vi "Set Target.vi"(6 "Axis":T1, 8 "error in (no error)":errorcluster, 9 "Target Rate Limit (T/min)":dbl, 10 "Target Field (T)":dbl[](array[numeric]), 11 "Instrument.VRM in":refnum<class "Instrument.OxfordVRM.lvclass">) -> (0 "error out":errorcluster, 2 "Response":string, 3 "Instrument.VRM out":refnum<class "Instrument.OxfordVRM.lvclass">)   [LabVIEW 2019, in "Instrument.OxfordVRM.lvclass"]
uses:
  Instrument.OxfordVRM.lvclass
  C:/Program Files (x86)/National Instruments/LabVIEW 2019/user.lib/LevyLab/Instrument Framework/SMOs/Instrument/Instrument.lvclass
  Typedefs/VRM Magnet Axis--Enum.ctl
  Typedefs/VRM Targets--Cluster.ctl
  Typedefs/Instrument.VRM.Commands-enum.ctl
  <userlib>/LevyLab/Instrument Framework/SMOs/Instrument/Instrument.lvclass/Instrument.ctl
  7bfbc778-14e2-498e-a779-e48ab3b8e301.vi
  7bfbc778-14e2-498e-a779-e48ab3b8e301.vi/26948dbf-a008-4a5f-8001-90938f97f5fa.vi
  7bfbc778-14e2-498e-a779-e48ab3b8e301.vi/26948dbf-a008-4a5f-8001-90938f97f5fa.vi/85d252fc-3981-4b1f-8816-d182b3c15b0a.vi
  <userlib>/LevyLab/Instrument Framework/SMOs/Instrument/API/Send and Receive.vi
  7bfbc778-14e2-498e-a779-e48ab3b8e301.vi/26948dbf-a008-4a5f-8001-90938f97f5fa.vi/d50f4601-6038-4c2c-b17e-43f1826cda29.vi
  <userlib>/LevyLab/Instrument Framework/SMOs/Instrument/Private/Get Client Type.vi
  7bfbc778-14e2-498e-a779-e48ab3b8e301.vi/26948dbf-a008-4a5f-8001-90938f97f5fa.vi/85d252fc-3981-4b1f-8816-d182b3c15b0a.vi/89440307-fee3-4c08-8f1d-a2867f85d077.vi
  7bfbc778-14e2-498e-a779-e48ab3b8e301.vi/26948dbf-a008-4a5f-8001-90938f97f5fa.vi/85d252fc-3981-4b1f-8816-d182b3c15b0a.vi/71707775-4b93-4dc6-a632-e85984a01861.vi
  7bfbc778-14e2-498e-a779-e48ab3b8e301.vi/26948dbf-a008-4a5f-8001-90938f97f5fa.vi/d50f4601-6038-4c2c-b17e-43f1826cda29.vi/ef93c44c-7e4a-41bd-a109-24ce89437007.vi
  7bfbc778-14e2-498e-a779-e48ab3b8e301.vi/26948dbf-a008-4a5f-8001-90938f97f5fa.vi/d50f4601-6038-4c2c-b17e-43f1826cda29.vi/b80f1979-f007-49e5-a589-a40ba76825d8.vi
  7bfbc778-14e2-498e-a779-e48ab3b8e301.vi/26948dbf-a008-4a5f-8001-90938f97f5fa.vi/d50f4601-6038-4c2c-b17e-43f1826cda29.vi/ef93c44c-7e4a-41bd-a109-24ce89437007.vi/5ddc282d-1542-424c-9eb1-353b70ff1e04.vi
  7bfbc778-14e2-498e-a779-e48ab3b8e301.vi/26948dbf-a008-4a5f-8001-90938f97f5fa.vi/d50f4601-6038-4c2c-b17e-43f1826cda29.vi/ef93c44c-7e4a-41bd-a109-24ce89437007.vi/fc9cd3dc-a458-4f07-8b6a-b3f87fbc8728.vi
  <userlib>/LevyLab/Instrument Framework/SMOs/Instrument/Private/Get RC Connection Status.vi
  <userlib>/LevyLab/Instrument Framework/SMOs/Instrument/API/Enum to String.vi
  <userlib>/LevyLab/Instrument Framework/SMOs/RemoteControl/API/Send and Receive.vi
  <vilib>/Utility/Data Type/Get Type Information.vi
  <vilib>/JDP Science/JSONtext/JSON text to Variant.vi
  <userlib>/LevyLab/Instrument Framework/SMOs/Instrument/API/Instrument.GetPublicEvents.vi
  <vilib>/JDP Science/JSONtext/Variant to JSON Text.vi
  <vilib>/National Instruments/GUID Generator/Guid Generator.vi
  <userlib>/LevyLab/Instrument Framework/SMOs/Instrument/API/Instrument.MessageToProcess.vi
  <userlib>/LevyLab/Instrument Framework/SMOs/Instrument/Private/Instrument.MessageFromProcess.EventStructure.vi
  <vilib>/JDP Science/JSONtext/LVClass Serializer/JSONtext LVClass Serializer.lvclass
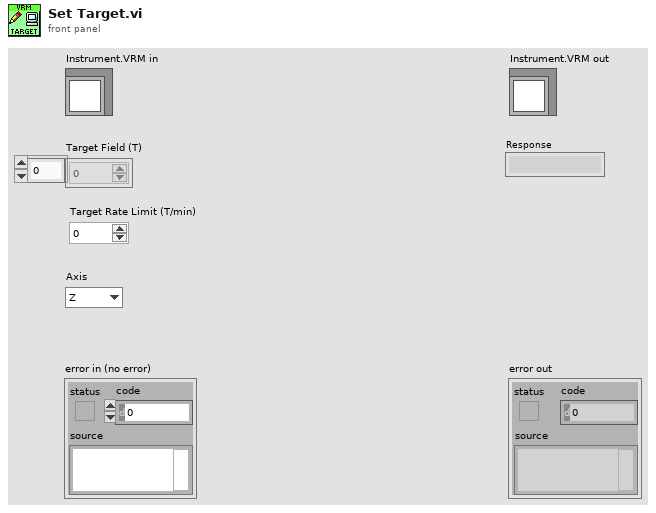
[diagram p1: front panel]
types:
  T1 = typedef "Instrument.OxfordVRM.lvclass/VRM Magnet Axis--Enum.ctl" = enum16{"Z", "X", "Y", "ALL"}
  T2 = typedef "Instrument.OxfordVRM.lvclass/Instrument.VRM.Commands-enum.ctl" = enum16{"setAction", "setTarget", "setMagnetField", "getStatus", "getTarget", "getMagnetField"}
  T3 = typedef "Instrument.OxfordVRM.lvclass/VRM Targets--Cluster.ctl" = cluster{"Field (T)":dbl[], "Field Rate (T/min)":dbl[], "Axis":T1}
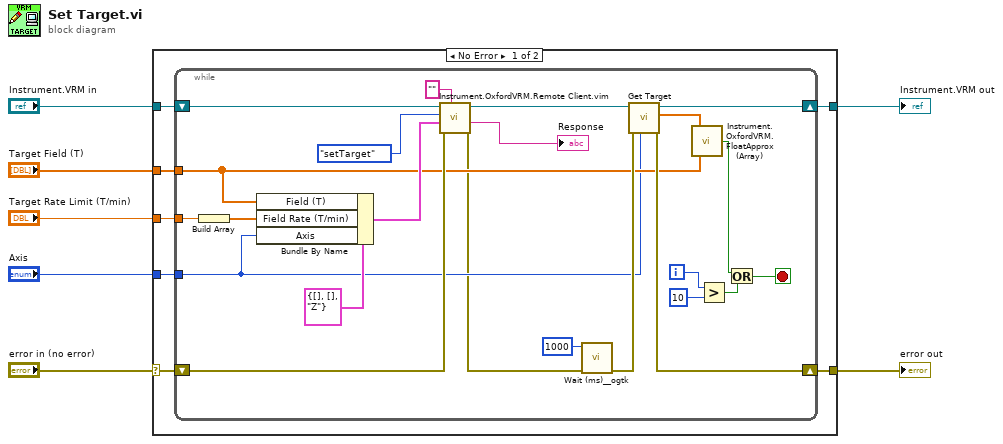
[diagram p0: block diagram]
diagram:
  n1 = case shown="No Error" "error in (no error)" {
    selector: "error in (no error)" -> [w11 w39]
    tunnel: "Target Rate Limit (T/min)" -> [w14 _]
    tunnel: [w9 w39] -> w6
    tunnel: "Target Field (T)" -> [w13 _]
    tunnel: "Instrument.VRM in" -> [w12 w38]
    tunnel: [w10 w38] -> w2
    tunnel: "Axis" -> [w8 _]
    frame No Error {
      n2 = while {
        tunnel: w14 -> [w16]
        tunnel: w13 -> [w24]
        shift-right: [w33] -> w10
        shift-left: w12 -> [w29]
        shift-right: [w32] -> w9
        shift-left: w11 -> [w34]
        tunnel: w8 -> [w22]
        i -> [w23]
        stop <- w26 stop-if-true
        n3 = Build Array(w16) -> (w15:dbl[])
        n4 = Bundle By Name(cluster=T3 {"Field (T)"=[], "Field Rate (T/min)"=[], "Axis"=enum."Z"} ("Mercury Targets"), "Field (T)"=w24, "Field Rate (T/min)"=w15, "Axis"=w22) -> (w35:T3)
        n5 = call "Instrument.OxfordVRM.Remote Client.vim"("Data Out type"="", "error in (no error)"=w34, "Data"=w35, "Commands"=Instrument.VRM.Commands-enum."setTarget", "Instrument.VRM in"=w29) -> ("error out"=w17:errorcluster, "Data out"=→"Response":string, "Instrument.VRM out"=w25:refnum<class "Instrument.OxfordVRM.lvclass">)  [unwired: 4 in]
        n6 = call <userlib>:"Wait (ms)__ogtk.vi"("error in (no error)"=w17, "milliseconds to wait"=u32 1000) -> ("error out"=w31:errorcluster)  [unwired: 8 in, 1 out]
        n7 = call "Get Target.vi"("Axis"=w22, "error in (no error)"=w31, "Instrument.VRM in"=w25) -> ("error out"=w32:errorcluster, "Target Field (T)"=w20:dbl[], "Instrument.VRM out"=w33:refnum<class "Instrument.OxfordVRM.lvclass">)  [unwired: 5 in, 1 out]
        n8 = call "Instrument.OxfordVRM.FloatApprox (Array).vi"("y"=w24, "x"=w20) -> ("x ~ y?"=w21:bool)  [unwired: 4 in]
        n9 = Greater?(x=w23, y=10) -> (0:w27:bool)
        n10 = Or(x=w21, y=w27) -> (x .or. y?=w26:bool)
      }
    }
    frame Error {
    }
  }
  "Instrument.VRM out" <- w2
  "error out" <- w6
